vi "BELLA PW scan mode shot control shutter.vi"(6 "ChF SCS off":dbl=0.006 caption="ChF no scan value" min=-9999999.0 max=9999999.0 format="%#_3f", 8 "error in (no error)":errorcluster, 9 "Expt editor SCS on":T1 {"Scan End" format="%#_6p"; "Scan Start" format="%#_6p"}, 10 "PostScanRate":dbl=0.006 min=-9999999.0 max=9999999.0 format="%#_3f", 11 "ScanShotControl":bool) -> (0 "error out":errorcluster, 3 "delay D to set":dbl)   [LabVIEW 2020]
uses:
  experiment editor scan delays SCS on off.ctl
  delay scan start and end.ctl
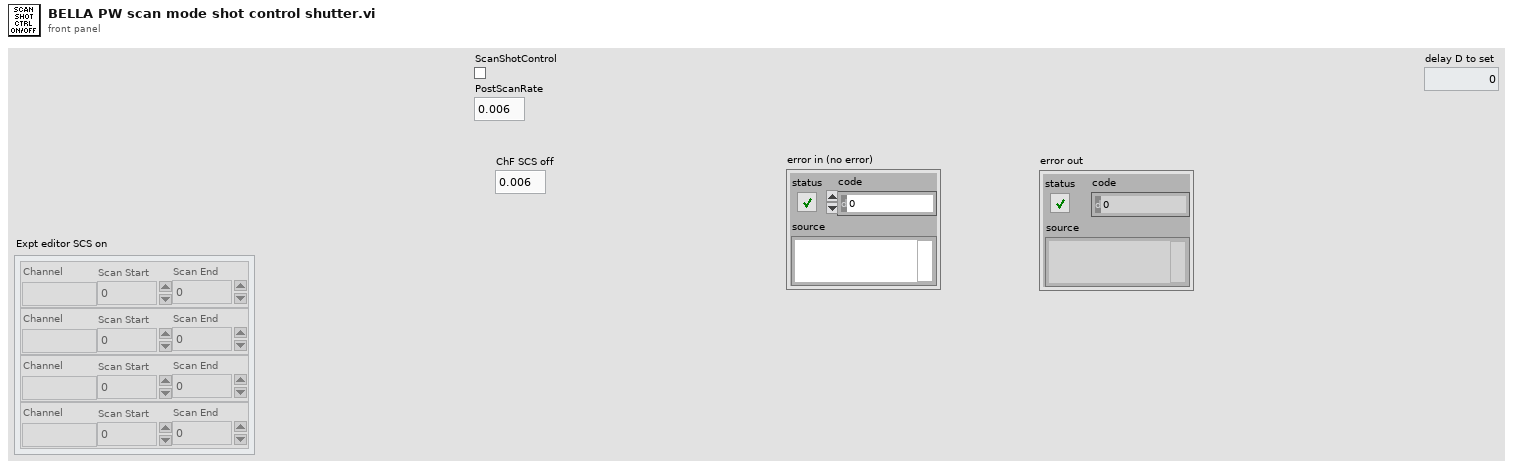
[diagram p1: front panel]
types:
  T1 = typedef "experiment editor scan delays SCS on off.ctl" = T2[]
  T2 = typedef "delay scan start and end.ctl" = cluster{"Channel":string, "Scan Start":dbl, "Scan End":dbl}
  T3 = typedef "mysql_authentication.ctl" = cluster{"User":string, "Password":string, "Database":string}
  T4 = cluster{"Port":u16, "IP Address":string, "Authentication":T3}
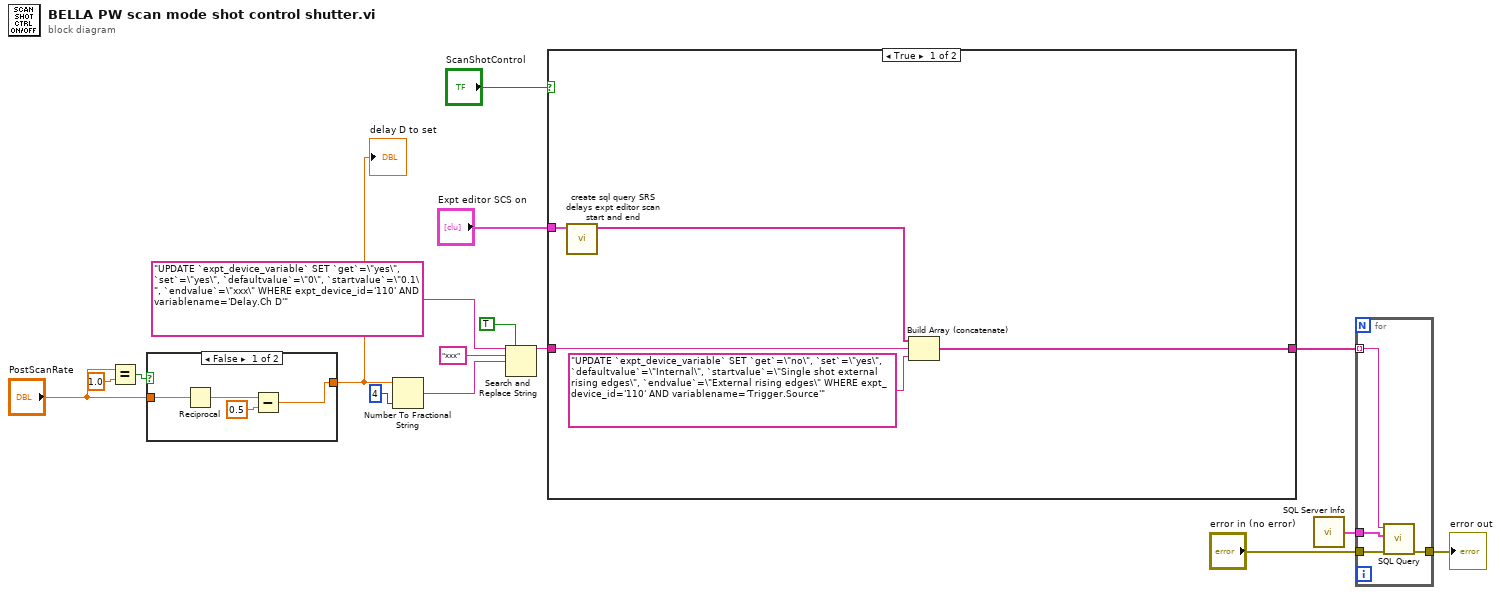
[diagram p0: block diagram]
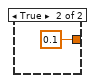
[diagram p2: hidden frame]
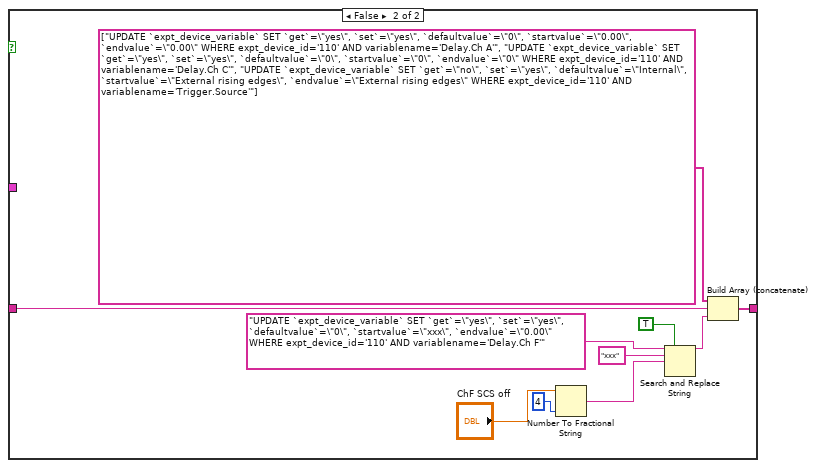
[diagram p3: hidden frame]
diagram:
  n1 = Equal?(x="PostScanRate", y=1.0) -> (x = y?=w9:bool)
  n2 = case shown="False" w9 {
    tunnel: "PostScanRate" -> [w20 _]
    tunnel: [w17 0.1 ("y")] -> w6
    frame False {
      n3 = Reciprocal(x=w20) -> (1/x=w19:dbl)
      n4 = Subtract(x=w19, y=0.5) -> (x-y=w17:dbl)
    }
    frame True {
    }
  }
  "delay D to set" <- w6
  n5 = Number To Fractional String(number=w6, precision (6)=i16 4) -> (F-format string=w8:string)  [unwired: 2 in]
  n6 = Search and Replace String(replace all?=TRUE ("replace all? (F)"), input string="UPDATE `expt_device_variable` SET `get`=\"yes\", `set`=\"yes\", `defaultvalue`=\"0\", `startvalue`=\"0.1\", `endvalue`=\"xxx\" WHERE expt_device_id='110' AND variablename='Delay.Ch D'" ("Query"), search string="xxx", replace string=w8) -> (result string=w2:string)  [unwired: 4 in, 3 out]
  n7 = case shown="True" "ScanShotControl" {
    tunnel: [w26 w35] -> w15
    tunnel: w2 -> [w25 w34]
    tunnel: "Expt editor SCS on" -> [w24 _]
    frame True {
      n8 = call "create sql query SRS delays expt editor scan start and end.vi"("Expt editor SCS on"=w24) -> ("Array"=w23:string[])  [unwired: 10 in]
      n9 = Build Array (concatenate)(w23, w25, "UPDATE `expt_device_variable` SET `get`=\"no\", `set`=\"yes\", `defaultvalue`=\"Internal\", `startvalue`=\"Single shot external rising edges\", `endvalue`=\"External rising edges\" WHERE expt_device_id='110' AND variablename='Trigger.Source'" ("Query")) -> (w26:string[])
    }
    frame False {
      n10 = Number To Fractional String(number="ChF SCS off", precision (6)=i16 4) -> (F-format string=w32:string)  [unwired: 2 in]
      n11 = Search and Replace String(replace all?=TRUE ("replace all? (F)"), input string="UPDATE `expt_device_variable` SET `get`=\"yes\", `set`=\"yes\", `defaultvalue`=\"0\", `startvalue`=\"xxx\", `endvalue`=\"0.00\" WHERE expt_device_id='110' AND variablename='Delay.Ch F'" ("Query"), search string="xxx", replace string=w32) -> (result string=w27:string)  [unwired: 4 in, 3 out]
      n12 = Build Array (concatenate)(string[] ["UPDATE `expt_device_variable` SET `get`=\"yes\", `set`=\"yes\", `defaultvalue`=\"0\", `startvalue`=\"0.00\", `endvalue`=\"0.00\" WHERE expt_device_id='110' AND variablename='Delay.Ch A'", "UPDATE `expt_device_variable` SET `get`=\"yes\", `set`=\"yes\", `defaultvalue`=\"0\", `startvalue`=\"0\", `endvalue`=\"0\" WHERE expt_device_id='110' AND variablename='Delay.Ch C'", "UPDATE `expt_device_variable` SET `get`=\"no\", `set`=\"yes\", `defaultvalue`=\"Internal\", `startvalue`=\"External rising edges\", `endvalue`=\"External rising edges\" WHERE expt_device_id='110' AND variablename='Trigger.Source'"], w34, w27) -> (w35:string[])
    }
  }
  n13 = call "SQL Server Info.vi"() -> ("SQL Server Info"=w16:T4)
  n14 = for {
    tunnel: w15 -> [w40] mode=indexing
    tunnel: w16 -> [w39]
    tunnel: "error in (no error)" -> [w38]
    tunnel: [w37] -> w12
    n15 = call "SQL Query.vi"("error in (no error)"=w38, "SQL Server Info"=w39, "Query"=w40) -> ("error out"=w37:errorcluster)  [unwired: 7 in, 1 out]
  }
  "error out" <- w12
